vi "N5700 Meas Output Current.vi"(5 "error":errorcluster, 8 "VISA":refnum<visa-resource-name>) -> (0 "error out":errorcluster, 2 "Output Current":dbl format="%.4f", 3 "VISA out":refnum<visa-resource-name>)   [LabVIEW 2020]
doc: "This VI returns the output current measured by the power supply (query \"MEAS:CURR?\")"
panel:
  # "Agilent Technologies  \nSeries N5700A\n  DC Power Supplies"
  # "Measure the \nOutput Current"
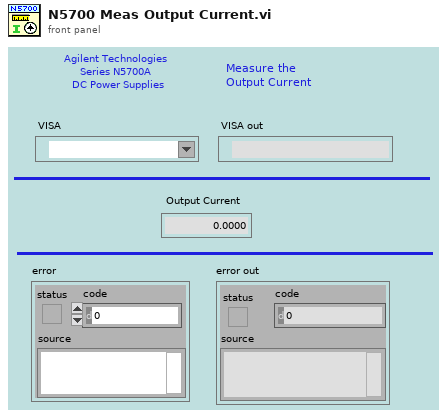
[diagram p1: front panel]
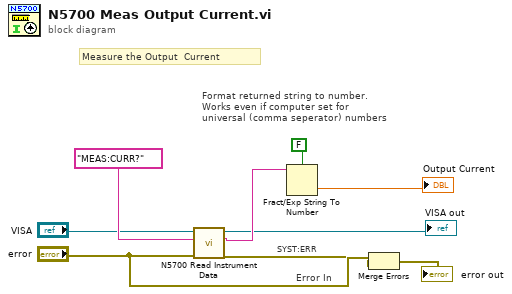
[diagram p0: block diagram]
diagram:
  # "SYST:ERR"
  # "Error In"
  # "Format returned string to number.\nWorks even if computer set for \nuniversal (comma seperator) numbers"
  # "Measure the Output  Current"
  n1 = call "N5700 Read Instrument Data.vi"("error"="error", "Query"="MEAS:CURR?" ("format string"), "VISA"="VISA") -> ("error out"=w1:errorcluster, "Response"=w6:string, "VISA out"=→"VISA out":refnum<visa-resource-name>)  [unwired: 2 in, 1 out]
  n2 = Fract/Exp String To Number(use system decimal point (T)=FALSE, string=w6) -> (number=→"Output Current":dbl)  [unwired: 2 in, 1 out]
  n3 = Merge Errors("error", w1) -> (→"error out":errorcluster)
